vi "updateNofPersons.vi"(0 "MySociety":refnum<class "HB_Society.lvclass">, 5 "error in (no error)":errorcluster) -> (14 "dup MySociety":refnum<class "HB_Society.lvclass">, 16 "nofPersons":dbl, 19 "error out":errorcluster)   [LabVIEW 2009, in "HB_BaseClass_Examples.lvlib" / "HB_Society.lvclass"]
doc: "Updates the sum of nofPersons of all Components of all hierarchies.\nEach whole in the hierarchie stores the sum of nofPersons of its own Components of all hierarchies below."
uses:
  HB_Society.lvclass
  HB_Society.lvclass/HB_Society.ctl
  lib.lib/HGF_LVC/HGF_BaseClasses/HGF_Composite/HGF_Composite.lvclass
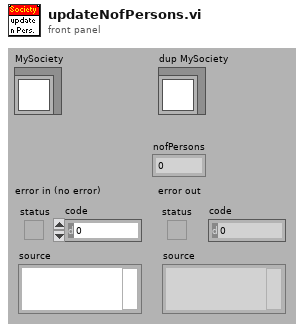
[diagram p1: front panel]
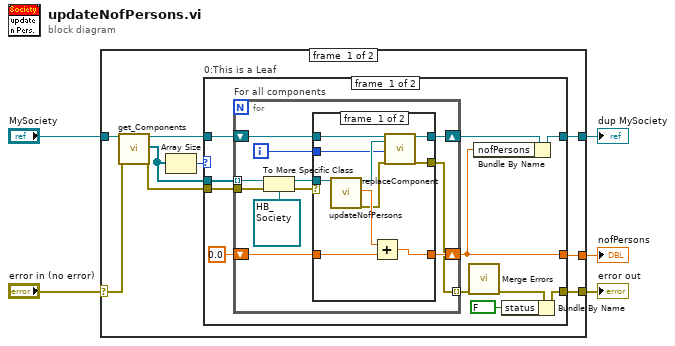
[diagram p0: block diagram]
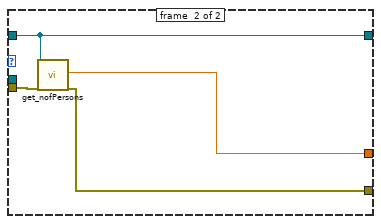
[diagram p3: hidden frame]
diagram:
  n1 = case shown="No Error" "error in (no error)" {
    selector: "error in (no error)" -> [w7 w54]
    tunnel: [w6 w54] -> w4
    tunnel: [w9 w55] -> w2
    tunnel: "MySociety" -> [w14 w55]
    tunnel: [w12 _] -> w1
    frame #0 {
      n2 = call "get_Components.vi"("HGF_Composite"=w14, "error in (no error)"=w7) -> ("dup HGF_Composite"=w10:refnum<class "HB_Society.lvclass">, "Components"=w11:refnum<class "HGF_Component.lvclass">[], "error out"=w8:errorcluster)  [unwired: 15 out]
      n3 = Array Size(array=w11) -> (size(s)=w13:i32)
      n4 = case "0:This is a Leaf" shown="0" w13 {
        tunnel: [w22 w52] -> w12
        tunnel: w10 -> [w20 w53]
        tunnel: w11 -> [w25 _]
        tunnel: [w23 w53] -> w9
        tunnel: w8 -> [w21 w51]
        tunnel: [w16 w50] -> w6
        frame #0 {
          n5 = for "For all components" {
            tunnel: w25 -> [w34] mode=indexing
            shift-right: [w32] -> w22
            shift-left: 0.0 -> [w33]
            tunnel: w21 -> [w31]
            shift-right: [w27] -> w19
            shift-left: w20 -> [w29]
            tunnel: [w26] -> w18 mode=indexing
            i -> [w28]
            n6 = To More Specific Class(target class=refnum<class "HB_Society.lvclass"> refnum ("MySociety.lvclass"), reference=w34, error in=w31) -> (specific class reference=w36:refnum<class "HB_Society.lvclass">, error out=w30:errorcluster)
            n7 = case shown="No Error" w30 {
              selector: w30 -> [_ w47]
              tunnel: w36 -> [w46 _]
              tunnel: w33 -> [w45 w49]
              tunnel: [w43 w49] -> w32
              tunnel: w29 -> [w42 w48]
              tunnel: w28 -> [w40 _]
              tunnel: [w39 w48] -> w27
              tunnel: [w37 w47] -> w26
              frame #0 {
                n8 = call-dynamic "updateNofPersons.vi"("MySociety"=w46) -> ("dup MySociety"=w41:refnum<class "HB_Society.lvclass">, "nofPersons"=w44:dbl, "error out"=w38:errorcluster)  [unwired: 1 in, 15 out]
                n9 = Add(x=w44, y=w45) -> (x+y=w43:dbl)
                n10 = call "replaceComponent.vi"("HGF_Composite"=w42, "HGF_Component"=w41, "objectIndex"=w40, "error in (no error)"=w38) -> ("dup HGF_Composite"=w39:refnum<class "HB_Society.lvclass">, "error out"=w37:errorcluster)  [unwired: 1 in, 13 out]
              }
              frame #1 {
              }
            }
          }
          n11 = call <vilib>:"Merge Errors.vi"("error array in"=w18) -> ("error out"=w17:errorcluster)  [unwired: 3 in, 3 out]
          n12 = Bundle By Name(cluster=w19, "nofPersons"=w22) -> (w23:refnum<class "HB_Society.lvclass">)
          n13 = Bundle By Name(cluster=w17, "status"=FALSE) -> (w16:errorcluster)
        }
        frame #1 {
          n14 = call "get_nofPersons.vi"("MySociety"=w53, "error in (no error)"=w51) -> ("nofPersons"=w52:dbl, "error out"=w50:errorcluster)  [unwired: 16 out]
        }
      }
    }
    frame #1 {
    }
  }
  "error out" <- w4
  "dup MySociety" <- w2
  "nofPersons" <- w1
